vi "ExCloseGlobalCam.vi"() -> ()   [LabVIEW 2012]
uses:
  CamHandle.vi
panel:
  out "Camera Closed":bool
  out "error out":errorcluster
  in  "error in (no error)":errorcluster
  # "ExCloseGlobalCam:\nThis vi closes a camera that is a global variable.  It will also\nfree any buffers allocated and unload toolkit dlls.\nThis vi MUST be run AFTER working with any vis that use the\nglobal camera handle."
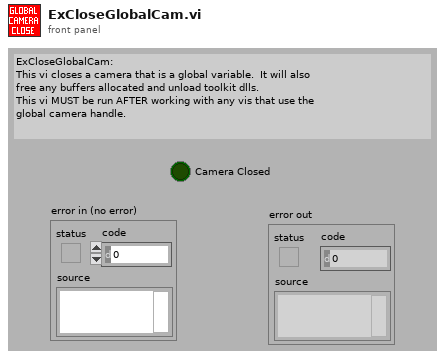
[diagram p1: front panel]
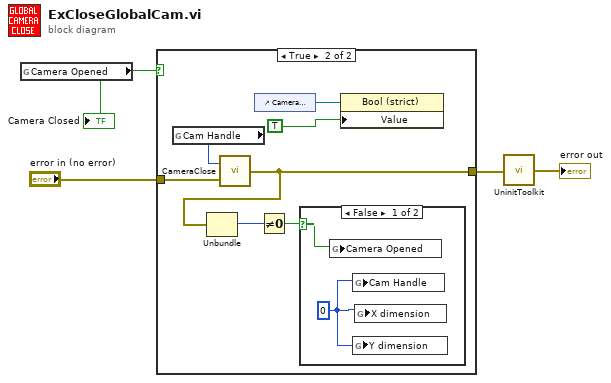
[diagram p0: block diagram]
diagram:
  n1 = global read "CamHandle.vi" "Camera Opened"() -> (w3:bool)
  "Camera Closed" <- w3
  n2 = case shown="True" w3 {
    tunnel: "error in (no error)" -> [w5 w12]
    tunnel: [w5 w7] -> w2
    frame False {
    }
    frame True {
      n3 = global read "CamHandle.vi" "Cam Handle"() -> (w11:u32)
      n4 = call <userlib>:"CameraClose.vi"("error in"=w12, "Camera Handle"=w11) -> ("error out"=w7:errorcluster)
      n5 = Unbundle(w7) -> ("code"=w9:i32)  [unwired: 2 out]
      n6 = control-ref of="Camera Closed"() -> (w10:refnum<vi>)
      n7 = Not Equal To 0?(x=w9) -> (x != 0?=w8:bool)
      n8 = case shown="False" w8 {
        selector: w8 -> [w14 _]
        frame False {
          w13 = 0
          n9 = global write "CamHandle.vi" "Camera Opened"(w14) -> ()
          n10 = global write "CamHandle.vi" "Cam Handle"(w13) -> ()
          n11 = global write "CamHandle.vi" "Y dimension"(w13) -> ()
          n12 = global write "CamHandle.vi" "X dimension"(w13) -> ()
        }
        frame True {
        }
      }
      n13 = property class="Bool (strict)"(reference=w10, "Value"=TRUE) -> ()  [unwired: 1 in, 2 out]
    }
  }
  n14 = call <userlib>:"UninitToolkit.vi"("error in"=w2) -> ("error out"=→"error out":errorcluster)
